vi "Periodic Tasks.vi"(8 "error in":errorcluster) -> ()   [LabVIEW 2018]
doc: "This VI runs in parallel to other tasks. It can contain as many user-defined periodic loops as you need. These can carry out PID or other sorts of timed response."
uses:
  <vilib>/Rock Robotics/WPI/ThirdParty/REV Robotics/SPARK MAX/Typedef/Spark MAX Faults.ctl
  <vilib>/Rock Robotics/WPI/ThirdParty/REV Robotics/SPARK MAX/Typedef/Spark MAX Limit Direction.ctl
  <vilib>/Rock Robotics/WPI/ThirdParty/REV Robotics/SPARK MAX/Typedef/Spark MAX Control Type.ctl
  <vilib>/Rock Robotics/WPI/Solenoid/WPI_SolenoidValue.ctl
  <vilib>/Rock Robotics/WPI/Utilities/WPI_GetSetVariantRefNum.vi
  <vilib>/Rock Robotics/WPI/Solenoid/WPI_SolenoidSetEnum.vi
  <vilib>/Rock Robotics/Network Tables/NT Write Boolean.vi
  <vilib>/Rock Robotics/Network Tables/NT Write Numeric Array.vi
  <vilib>/Rock Robotics/Network Tables/NT Write Boolean Array.vi
  <vilib>/Rock Robotics/Network Tables/NT Read Number.vi
  <vilib>/Rock Robotics/Network Tables/NT Write Number.vi
  <vilib>/addons/control/pid/pid.llb/PID (DBL).vi
  <vilib>/Rock Robotics/WPI/Solenoid/WPI_SolenoidGetEnum.vi
  <vilib>/addons/control/pid/NI_PID_pid.lvlib
panel:
  in  "setpoint":dbl format="%.2f"
  in  "cargoship":dbl=3.0 format="%#_13g"
  in  "rocket":dbl=4.699999999999999 format="%#_13g"
  in  "intake":dbl=10.65 format="%#_13g"
  out "Current":dbl=0.125
  out "Applied Output":dbl
  out "Set Point":i32=4
  out "x":dbl
  out "angle":dbl
  in  "PID Constants":T1={"P Gain"=0.08, "I Gain"=7e-05, "D Gain"=2.0, "F Gain"=0.0, "I Zone"=4.0, "Min Output"=-0.2, "Max Output"=0.05}
  in  "PID gains":T2={"proportional gain (Kc)"=0.01, "integral time (Ti, min)"=0.006, "derivative time (Td, min)"=0.0} {"derivative time (Td, min)" format="%.3f"; "integral time (Ti, min)" format="%.3f"; "proportional gain (Kc)" format="%.3f"}
  out "output":dbl=0.041618055988639956 format="%.2f"
  out "Direction":bool
  out "Turret Encoder":dbl=0.75
  out "Faults":T3={"Hard Limit Rev"=FALSE, "Hard Limit Fwd"=TRUE, "Soft Limit Fwd"=FALSE, "Soft Limit Rev"=FALSE, "Other Fault"=FALSE, "DRV Fault"=FALSE, "Has Reset?"=FALSE, "CAN RX"=FALSE, "CAN TX"=FALSE, "EEPROM CRC"=FALSE, "Stall"=FALSE, "Sensor Fault"=FALSE, "Motor Type Fault"=FALSE, "IWDT Reset"=FALSE, "Over Current"=FALSE, "Brownout"=FALSE}
  out "Sticky Faults":T3={"Hard Limit Rev"=FALSE, "Hard Limit Fwd"=FALSE, "Soft Limit Fwd"=FALSE, "Soft Limit Rev"=FALSE, "Other Fault"=FALSE, "DRV Fault"=FALSE, "Has Reset?"=FALSE, "CAN RX"=FALSE, "CAN TX"=TRUE, "EEPROM CRC"=FALSE, "Stall"=FALSE, "Sensor Fault"=FALSE, "Motor Type Fault"=FALSE, "IWDT Reset"=FALSE, "Over Current"=FALSE, "Brownout"=FALSE}
  out "Left Motor RPM":dbl
  out "Left Motor Rotations":dbl=10.976247787475586 format="%#_6p"
  # "SPARX MAX/ARM"
  # "SPARX/TURRET"
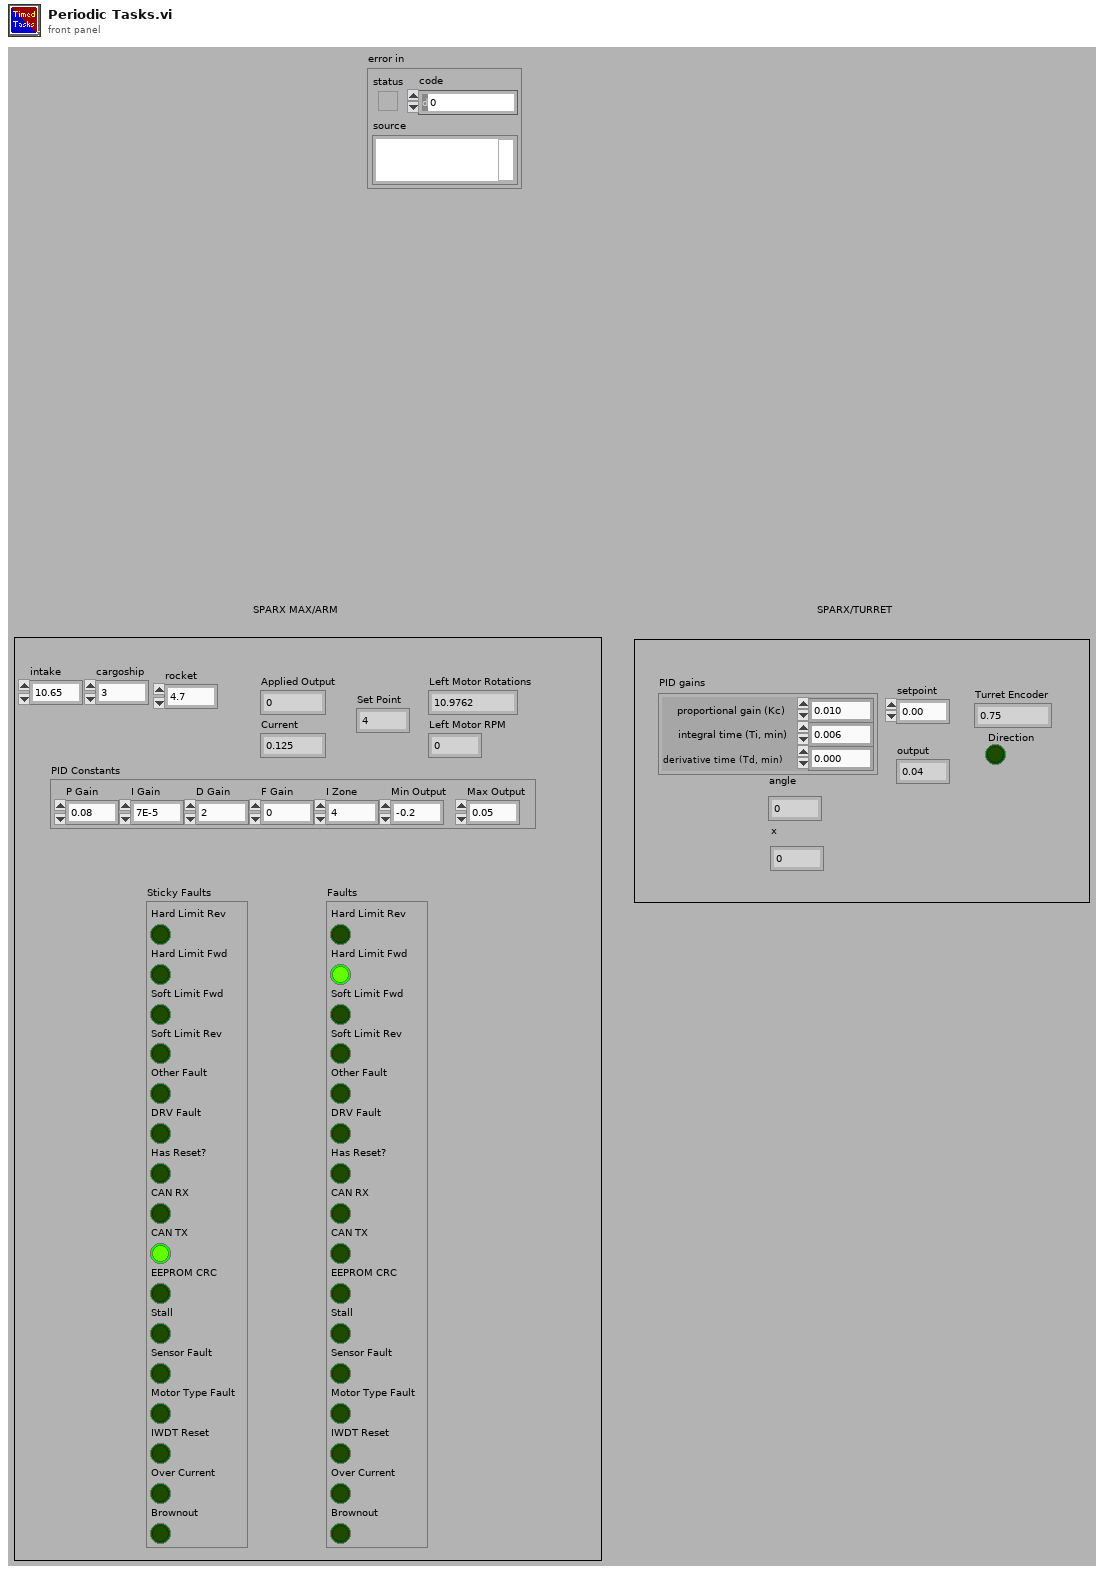
[diagram p1: front panel]
types:
  T1 = cluster{"P Gain":dbl, "I Gain":dbl, "D Gain":dbl, "F Gain":dbl, "I Zone":dbl, "Min Output":dbl, "Max Output":dbl}
  T2 = cluster{"proportional gain (Kc)":dbl, "integral time (Ti, min)":dbl, "derivative time (Td, min)":dbl}
  T3 = typedef "Spark MAX Faults.ctl" = cluster{"Hard Limit Rev":bool, "Hard Limit Fwd":bool, "Soft Limit Fwd":bool, "Soft Limit Rev":bool, "Other Fault":bool, "DRV Fault":bool, "Has Reset?":bool, "CAN RX":bool, "CAN TX":bool, "EEPROM CRC":bool, "Stall":bool, "Sensor Fault":bool, "Motor Type Fault":bool, "IWDT Reset":bool, "Over Current":bool, "Brownout":bool}
  T4 = typedef "WPI_JoystickDevRef.ctl" = cluster{"Device":T5}
  T5 = typedef "WPI_JoystickDeviceEnum.ctl" = enum16{"USB 0", "USB 1", "USB 2", "USB 3", "USB 4", "USB 5"}
  T6 = typedef "WPI_RobotDriveDevRef.ctl" = cluster{"DevStatus":errorcluster, "Motors[]":T7[], "Square Inputs":bool, "Max Output":dbl}
  T7 = typedef "WPI_MotorControlDeviceRef.ctl" = cluster{"DeviceStatus":errorcluster, "Type":T8, "PWM":cluster{"PWM Channel":T9, "DeadBand":T10}, "CAN":cluster{"Device Number":u8, "SetOutput VI Ref":variant, "GetOutput VI Ref":variant, "Enable VI Ref":variant, "Disable VI Ref":variant, "Data":variant}, "Invert":bool, "DIO PWM":cluster{"PWM \"Enable\" Channel":T9, "DIOChannel":T11, "PWM Rate":dbl}}
  T8 = typedef "WPI_MotorControlType.ctl" = enum16{"PWM", "CAN", "DIO PWM"}
  T9 = typedef "FPGA_DIOPWMChannel.ctl" = enum8{"PWM 0", "PWM 1", "PWM 2", "PWM 3", "PWM 4", "PWM 5", "PWM 6", "PWM 7", "PWM 8", "PWM 9", "PWM MXP 0", "PWM MXP 1", "PWM MXP 2", "PWM MXP 3", "PWM MXP 4", "PWM MXP 5", "PWM MXP 6", "PWM MXP 7", "PWM MXP 8", "PWM MXP 9", "Invalid"}
  T10 = typedef "WPI_PWMDeadband.ctl" = cluster{"Name":string, "maxPositivePwm":i32, "minPositivePwm":i32, "centerPwm":i32, "maxNegativePwm":i32, "minNegativePwm":i32, "angularRange":u16}
  T11 = typedef "FPGA_DIOChannel.ctl" = enum8{"DIO 0", "DIO 1", "DIO 2", "DIO 3", "DIO 4", "DIO 5", "DIO 6", "DIO 7", "DIO 8", "DIO 9", "DIO MXP 0", "DIO MXP 1", "DIO MXP 2", "DIO MXP 3", "DIO MXP 4", "DIO MXP 5", "DIO MXP 6", "DIO MXP 7", "DIO MXP 8", "DIO MXP 9", "DIO MXP 10", "DIO MXP 11", "DIO MXP 12", "DIO MXP 13", "DIO MXP 14", "DIO MXP 15", "SPI Port CS1", "SPI Port CS2", "SPI Port CS3", "SPI Port MISO", "SPI Port MOSI", "Invalid"}
  T12 = typedef "Spark MAX Control Type.ctl" = enum16{"Percent VBus", "Voltage", "Velocity", "Position", "Smart Motion", "Current", "Smart Velocity"}
  T13 = typedef "Spark MAX Limit Direction.ctl" = enum16{"Forward Limit", "Reverse Limit"}
  T14 = typedef "WPI_EncoderDevRef.ctl" = cluster{"DevStatus":errorcluster, "EncoderIndex":T15, "CounterIndex":T16, "DistancePerCount":dbl, "Decoding Type":T17}
  T15 = typedef "FPGA_EncoderIdx.ctl" = enum8{"Enc 0", "Enc 1", "Enc 2", "Enc 3", "Enc 4", "Enc 5", "Enc 6", "Enc 7", "Invalid"}
  T16 = typedef "FPGA_CounterCtrSystemIndex.ctl" = enum8{"Ctr 0", "Ctr 1", "Ctr 2", "Ctr 3", "Ctr 4", "Ctr 5", "Ctr 6", "Ctr 7", "Invalid"}
  T17 = typedef "WPI_EncoderType.ctl" = enum16{"1x", "2x", "4x"}
  T18 = typedef "WPI_SwitchDevRef.ctl" = cluster{"DevStatus":errorcluster, "DIO Channel":T11, "CntIndex":T16, "Normally Closed":bool}
  T19 = typedef "WPI_SolenoidValue.ctl" = enum16{"Off", "On", "Forward", "Reverse"}
  T20 = typedef "WPI_SolenoidDevRef.ctl" = cluster{"DevStatus":errorcluster, "Pneumatics Control Module":u8, "Forward Solenoid Channel":T21, "Reverse Solenoid Channel":T21}
  T21 = typedef "WPI_SolenoidChannel.ctl" = enum8{"Solenoid 0", "Solenoid 1", "Solenoid 2", "Solenoid 3", "Solenoid 4", "Solenoid 5", "Solenoid 6", "Solenoid 7", "Invalid"}
  T22 = typedef "WPI_DigitalInputDevRef.ctl" = cluster{"DevStatus":errorcluster, "DIO Channel":T11}
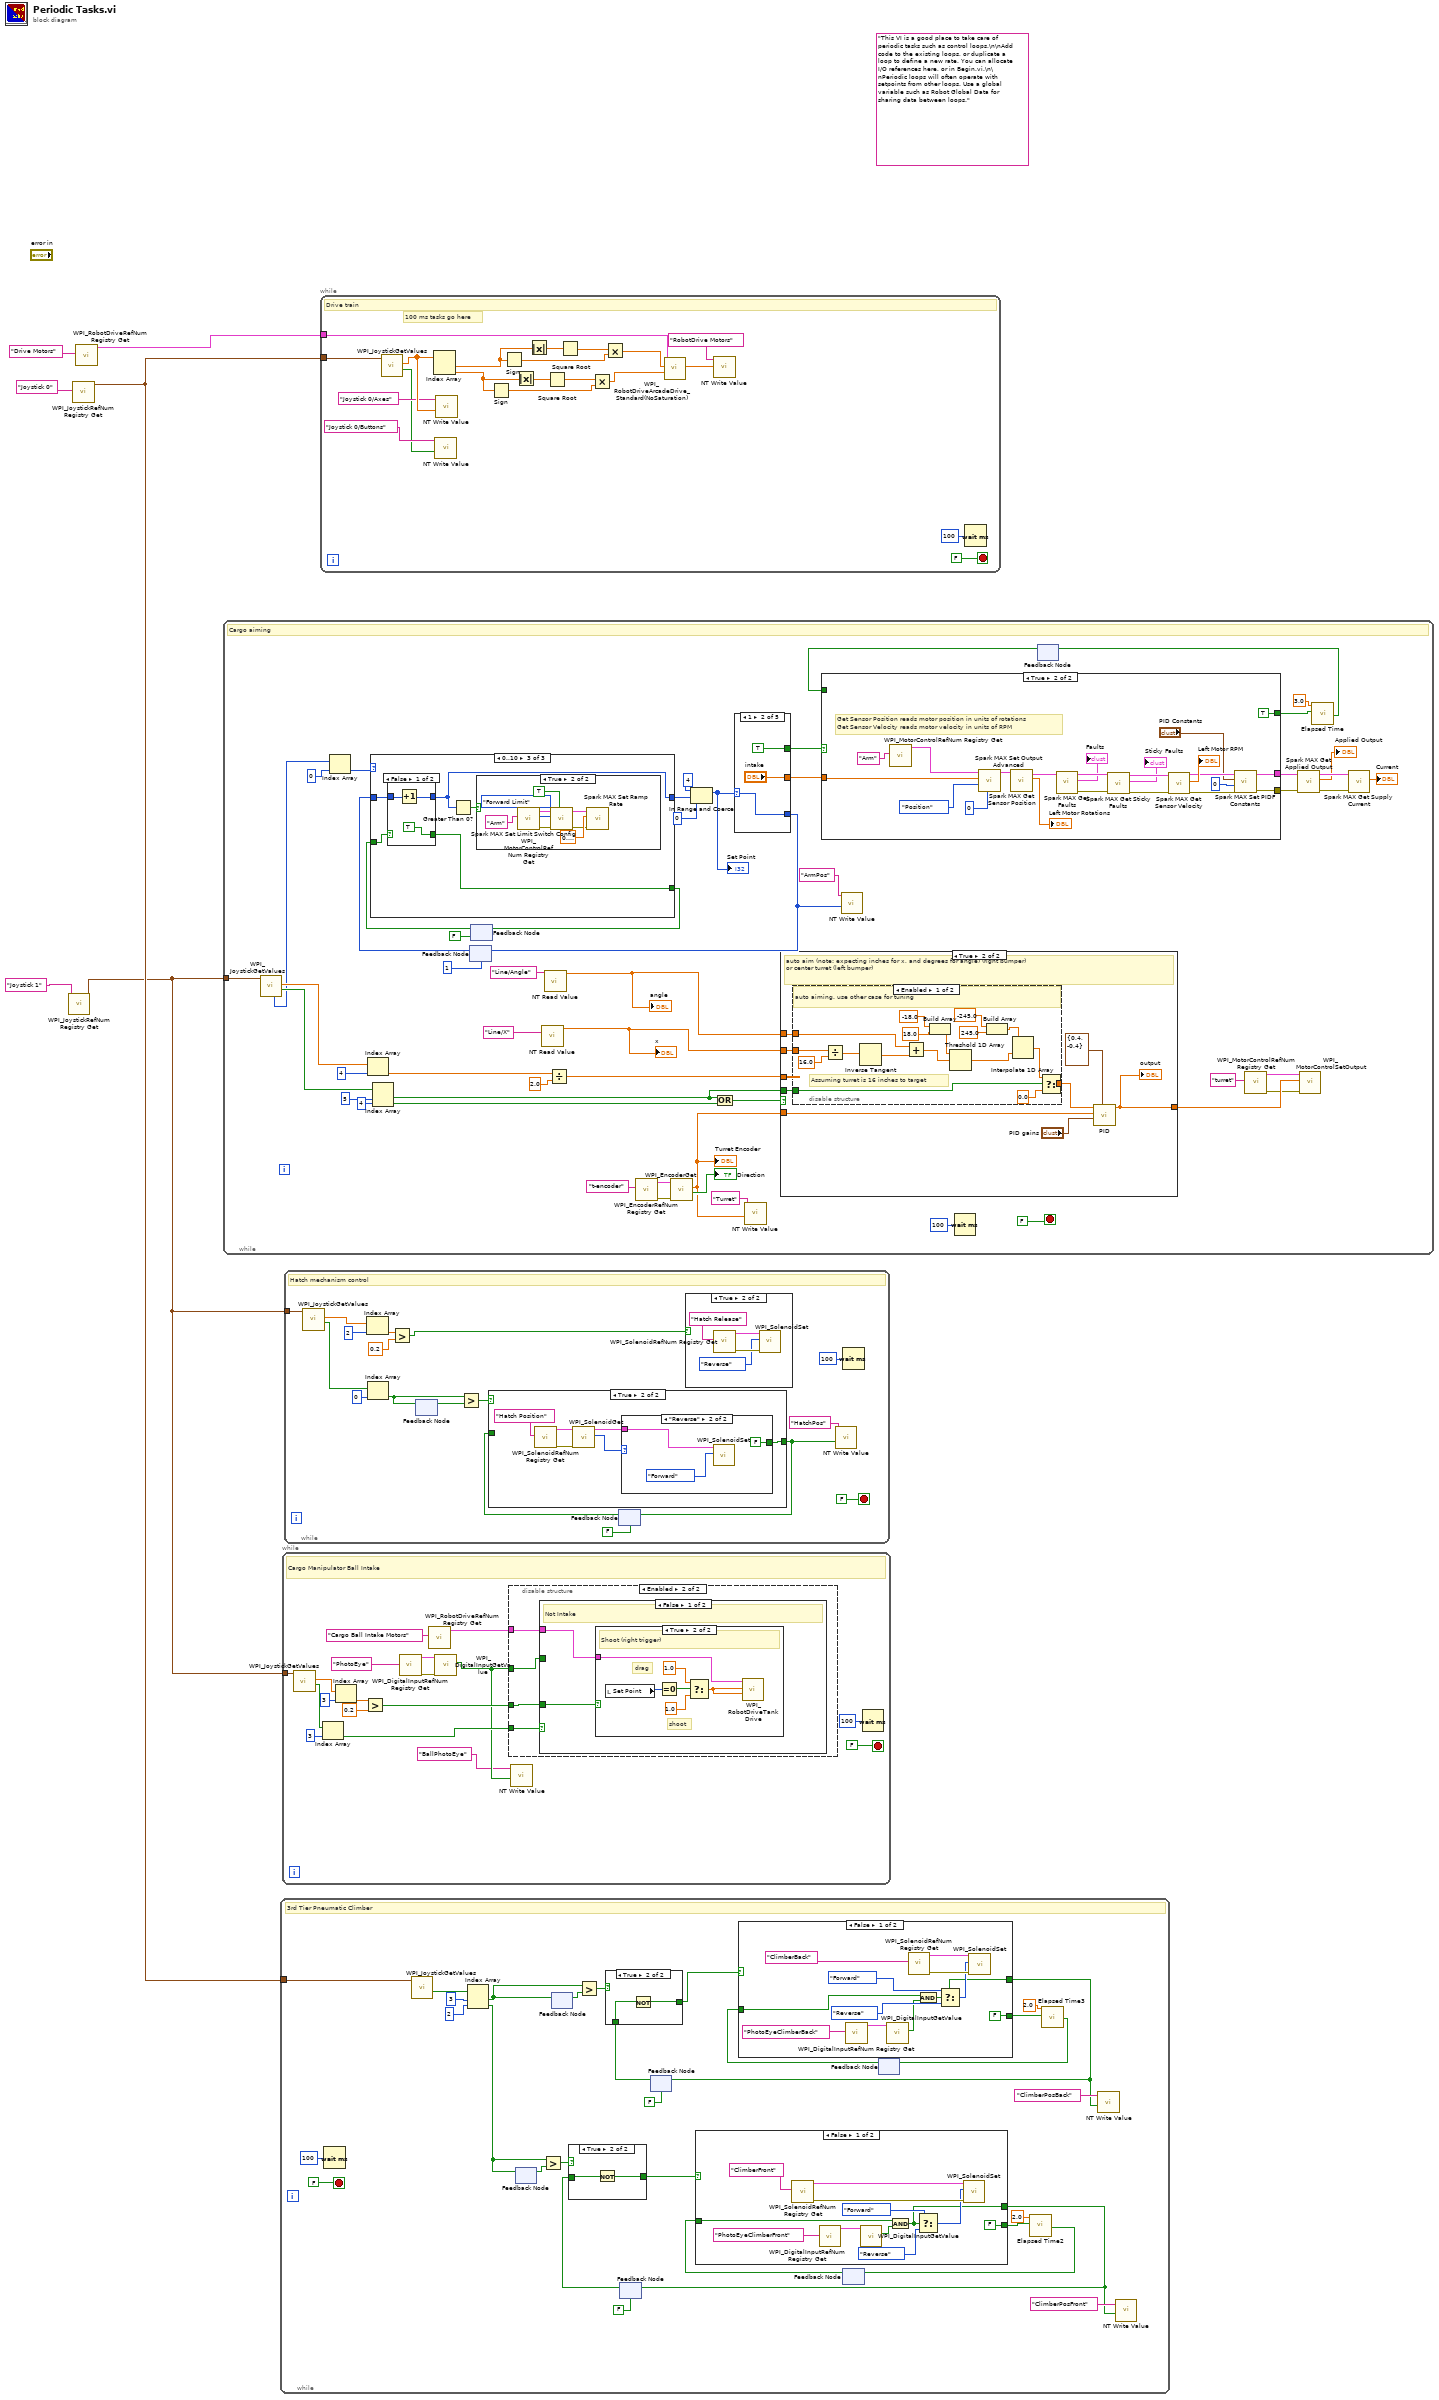
[diagram p0: block diagram]
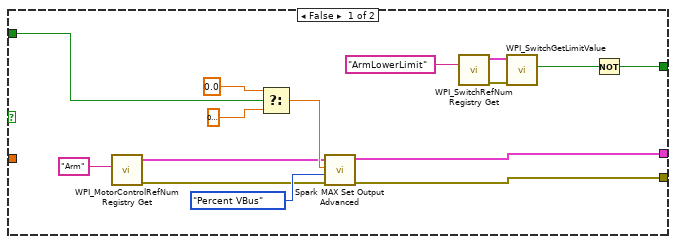
[diagram p2: hidden frame]
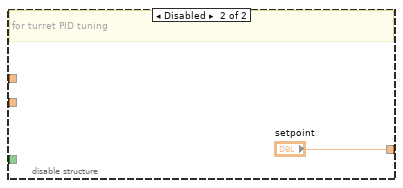
[diagram p4: hidden frame]
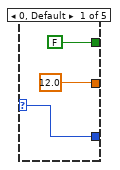
[diagram p5: hidden frame]
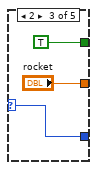
[diagram p6: hidden frame]
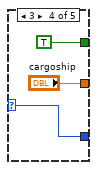
[diagram p7: hidden frame]
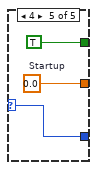
[diagram p8: hidden frame]
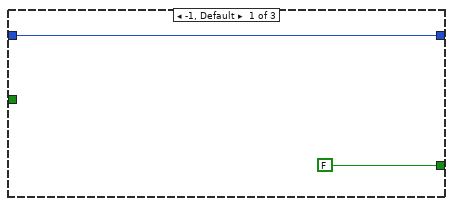
[diagram p9: hidden frame]
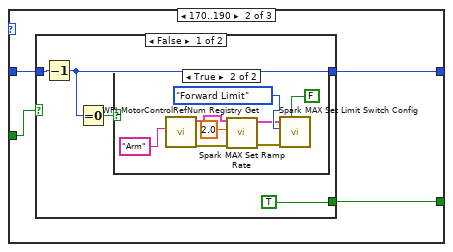
[diagram p10: hidden frame]
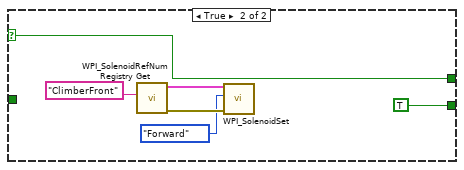
[diagram p16: hidden frame]
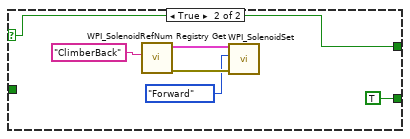
[diagram p18: hidden frame]
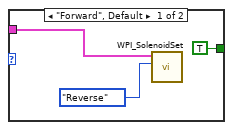
[diagram p20: hidden frame]
diagram:
  (unwired) "This VI is a good place to take care of periodic tasks such as control loops.\n\nAdd code to the existing loops, or duplicate a loop to define a new rate. You can allocate I/O references here, or in Begin.vi.\n\nPeriodic loops will often operate with setpoints from other loops. Use a global variable such as Robot Global Data for sharing data between loops."
  n1 = call <vilib>:"WPI_JoystickRefNum Registry Get.vi"("refnum name"="Joystick 1") -> ("JoystickDevRef"=w1:T4)  [unwired: 1 in, 9 out]
  n2 = call <vilib>:"WPI_JoystickRefNum Registry Get.vi"("refnum name"="Joystick 0") -> ("JoystickDevRef"=w2:T4)  [unwired: 1 in, 9 out]
  n3 = call <vilib>:"WPI_RobotDriveRefNum Registry Get.vi"("refnum name"="Drive Motors") -> ("RobotDriveDevRef"=w4:T6)  [unwired: 1 in, 9 out]
  n4 = while {
    tunnel: w1 -> [w54]
    stop <- FALSE stop-if-true
    # "Cargo aiming"
    n5 = call <vilib>:"WPI_JoystickGetValues.vi"("JoystickDevRef"=w54) -> ("Buttons"=w51:bool[], "Axes"=w53:dbl[], "POVs"=w47:i16[])  [unwired: 6 in, 2 out]
    n6 = Index Array(array=w47, index=0) -> (element=w45:i16)
    n7 = Index Array(array=w53, index=4) -> (element=w42:dbl)
    n8 = Index Array(array=w51, index #1=5 ("index"), index #2=4 ("index")) -> (element #1=w22:bool, element #2=w23:bool)
    n9 = feedback #1(1) -> (w44:i32)
    n10 = feedback #2(FALSE) -> (w28:bool)
    n11 = case shown="0..10" w45 {
      tunnel: w28 -> [_ w143 w163]
      tunnel: [FALSE w142 w162] -> w29
      tunnel: w44 -> [w140 w145 w164]
      tunnel: [w140 w144 w161] -> w27
      frame -1, Default {
      }
      frame 170..190 {
        n12 = case shown="False" w143 {
          selector: w143 -> [_ w158]
          tunnel: w145 -> [w149 w159]
          tunnel: [w146 w159] -> w144
          tunnel: [TRUE w158] -> w142
          frame False {
            n13 = Decrement(x=w149) -> (x-1=w146:i32)
            n14 = Equal To 0?(x=w146) -> (x = 0?=w147:bool)
            n15 = case shown="True" w147 {
              frame False {
              }
              frame True {
                n16 = call <vilib>:"WPI_MotorControlRefNum Registry Get.vi"("refnum name"="Arm") -> ("error out"=w150:errorcluster, "MotorControlDevRef"=w153:T7)  [unwired: 9 in]
                n17 = call <vilib>:"Spark MAX Set Ramp Rate.vi"("error in (no error)"=w150, "Seconds from neutral to full (0)"=sgl 2.0, "MotorControlDeviceRef in"=w153) -> ("error out"=w151:errorcluster, "MotorControlDeviceRef"=w152:T7)  [unwired: 7 in]
                n18 = call <vilib>:"Spark MAX Set Limit Switch Config.vi"("Enabled? (T)"=FALSE, "error in (no error)"=w151, "Limit Switch"=Spark_MAX_Limit_Direction."Forward Limit", "MotorControlDeviceRef in"=w152) -> ()  [unwired: 6 in, 2 out]
              }
            }
          }
          frame True {
          }
        }
      }
      frame 0..10 {
        n19 = case shown="False" w163 {
          selector: w163 -> [_ w177]
          tunnel: w164 -> [w175 w176]
          tunnel: [w174 w176] -> w161
          tunnel: [TRUE w177] -> w162
          frame False {
            n20 = Increment(x=w175) -> (x+1=w174:i32)
          }
          frame True {
          }
        }
        n21 = Greater Than 0?(x=w161) -> (x > 0?=w160:bool)
        n22 = case shown="True" w160 {
          frame False {
          }
          frame True {
            n23 = call <vilib>:"WPI_MotorControlRefNum Registry Get.vi"("refnum name"="Arm") -> ("error out"=w171:errorcluster, "MotorControlDevRef"=w170:T7)  [unwired: 9 in]
            n24 = call <vilib>:"Spark MAX Set Limit Switch Config.vi"("Enabled? (T)"=TRUE, "error in (no error)"=w171, "Limit Switch"=Spark_MAX_Limit_Direction."Forward Limit", "MotorControlDeviceRef in"=w170) -> ("error out"=w166:errorcluster, "MotorControlDeviceRef out"=w165:T7)  [unwired: 6 in]
            n25 = call <vilib>:"Spark MAX Set Ramp Rate.vi"("error in (no error)"=w166, "Seconds from neutral to full (0)"=sgl 0.1, "MotorControlDeviceRef in"=w165) -> ()  [unwired: 7 in, 2 out]
          }
        }
      }
    }
    n26 = feedback-in #2(w29) -> ()
    n27 = call-poly <vilib>:"NT Read Value.vi"("Name"="Line/X") -> ("Numeric"=w10:dbl)  [unwired: 9 in, 1 out]
    "x" <- w10
    n28 = call-poly <vilib>:"NT Read Value.vi"("Name"="Line/Angle") -> ("Numeric"=w9:dbl)  [unwired: 9 in, 1 out]
    "angle" <- w9
    n29 = Divide(x=w42, y=2.0) -> (x/y=w33:dbl)
    n30 = call <vilib>:"WPI_EncoderRefNum Registry Get.vi"("refnum name"="t-encoder") -> ("error out"=w59:errorcluster, "EncoderDevRef"=w58:T14)  [unwired: 9 in]
    n31 = call <vilib>:"WPI_EncoderGet.vi"("error in (no error)"=w59, "EncoderDevRef"=w58) -> ("Direction"=→"Direction":bool, "Distance"=w7:dbl)  [unwired: 4 in, 4 out]
    "Turret Encoder" <- w7
    n32 = In Range and Coerce(upper limit=4, x=w27, lower limit=0) -> (coerced(x)=w25:i32)  [unwired: 1 out]
    "Set Point" <- w25
    n33 = Or(x=w22, y=w23) -> (x .or. y?=w24:bool)
    n34 = case shown="1" w25 {
      selector: w25 -> [w127 w129 w132 w135 w138]
      tunnel: [12.0 "intake" "rocket" "cargoship" w139] -> w41
      tunnel: [w127 w129 w132 w135 w138] -> w38
      tunnel: [FALSE TRUE TRUE TRUE TRUE] -> w40
      frame 0, Default {
      }
      frame 1 {
      }
      frame 2 {
      }
      frame 3 {
      }
      frame 4 {
        w139 = 0.0  # Startup
      }
    }
    n35 = feedback-in #1(w38) -> ()
    n36 = call-poly <vilib>:"NT Write Value.vi"("Numeric"=w7, "Name"="Turret") -> ()  [unwired: 9 in, 1 out]
    n37 = case shown="True" w24 {
      tunnel: w9 -> [_ w101]
      tunnel: w10 -> [_ w102]
      tunnel: w33 -> [w98 _]
      tunnel: [w98 w103] -> w39
      tunnel: w7 -> [_ w104]
      tunnel: w22 -> [_ w100]
      frame False {
        # "manual control"
      }
      frame True {
        # "auto aim (note: expecting inches for x, and degrees for angle) (right bumper)\nor center turret (left bumper)"
        n38 = disable-structure shown="Enabled" {
          disable-tunnel: w102 -> [w123 _]
          disable-tunnel: w101 -> [w121 _]
          disable-tunnel: w100 -> [w108 _]
          disable-tunnel: [w107 "setpoint"] -> w99
          frame Enabled {
            # "Assuming turret is 16 inches to target"
            # "auto aiming. use other case for tuning"
            n39 = Divide(x=w123, y=16.0) -> (x/y=w112:dbl)
            n40 = Inverse Tangent(1:w112) -> (0:w111:dbl)
            n41 = Add(x=w121, y=w111) -> (x+y=w115:dbl)
            n42 = Build Array(-18.0 ("lower limit"), 18.0 ("upper limit")) -> (w116:dbl[])
            n43 = Threshold 1D Array(2:w115, 3:w116) -> (0:w113:dbl)  [unwired: 1 in]
            n44 = Build Array(-245.0 ("lower limit"), 245.0 ("upper limit")) -> (w114:dbl[])
            n45 = Interpolate 1D Array(1:w113, 2:w114) -> (0:w110:dbl)
            n46 = Select(t=w110, s=w108, f=0.0) -> (s? t:f=w107:dbl)
          }
          frame Disabled {
            # "for turret PID tuning"
          }
        }
        n47 = call-poly <vilib>:"PID.vi"("output range"=cluster{"output high":dbl, "output low":dbl} {"output high"=0.4, "output low"=-0.4}, "PID gains"="PID gains", "process variable"=w104, "setpoint"=w99) -> ("output"=w103:dbl)  [unwired: 6 in, 1 out]
        "output" <- w103
      }
    }
    n48 = call-poly <vilib>:"NT Write Value.vi"("Numeric"=w38, "Name"="ArmPos") -> ()  [unwired: 9 in, 1 out]
    n49 = Wait (ms)(milliseconds to wait=u32 100) -> ()  [unwired: 1 out]
    n50 = feedback #3() -> (w12:bool)  [unwired: 1 in]
    n51 = case shown="True" w40 {
      tunnel: w41 -> [_ w79]
      tunnel: [w68 w77] -> w16
      tunnel: [w67 w78] -> w15
      tunnel: w12 -> [w66 _]
      tunnel: [w65 TRUE] -> w11
      frame False {
        n52 = call <vilib>:"WPI_MotorControlRefNum Registry Get.vi"("refnum name"="Arm") -> ("error out"=w69:errorcluster, "MotorControlDevRef"=w70:T7)  [unwired: 9 in]
        n53 = Select(t=0.0, s=w66, f=0.9999999999999999 ("Setpoint")) -> (s? t:f=w71:dbl)
        n54 = call <vilib>:"Spark MAX Set Output Advanced.vi"("error in (no error)"=w69, "Control Mode"=Spark_MAX_Control_Type."Percent VBus", "Setpoint"=w71, "MotorControlDevRef"=w70) -> ("error out"=w68:errorcluster, "MotorControlDevRef"=w67:T7)  [unwired: 6 in]
        n55 = call <vilib>:"WPI_SwitchRefNum Registry Get.vi"("refnum name"="ArmLowerLimit") -> ("error out"=w63:errorcluster, "SwitchDevRef"=w64:T18)  [unwired: 9 in]
        n56 = call <vilib>:"WPI_SwitchGetLimitValue.vi"("error in (no error)"=w63, "SwitchDevRef"=w64) -> ("Switch Pressed"=w61:bool)  [unwired: 7 in, 2 out]
        n57 = Not(x=w61) -> (.not. x?=w65:bool)
      }
      frame True {
        # "Get Sensor Position reads motor position in units of rotations\nGet Sensor Velocity reads motor velocity in units of RPM"
        n58 = call <vilib>:"WPI_MotorControlRefNum Registry Get.vi"("refnum name"="Arm") -> ("MotorControlDevRef"=w81:T7)  [unwired: 9 in, 1 out]
        n59 = call <vilib>:"Spark MAX Set Output Advanced.vi"("PIDF Slot (0)"=0, "Control Mode"=Spark_MAX_Control_Type."Position", "Setpoint"=w79, "MotorControlDevRef"=w81) -> ("MotorControlDevRef"=w95:T7)  [unwired: 6 in, 1 out]
        n60 = call <vilib>:"Spark MAX Get Sensor Position.vi"("MotorControlDevRef in"=w95) -> ("Sensor Position"=→"Left Motor Rotations":dbl, "MotorControlDevRef out"=w93:T7)  [unwired: 7 in, 2 out]
        n61 = call <vilib>:"Spark MAX Get Faults.vi"("MotorControlDevRef in"=w93) -> ("error out"=w92:errorcluster, "Faults"=→"Faults":T3, "MotorControlDevRef out"=w91:T7)  [unwired: 7 in, 1 out]
        n62 = call <vilib>:"Spark MAX Get Sticky Faults.vi"("error in (no error)"=w92, "MotorControlDevRef in"=w91) -> ("error out"=w89:errorcluster, "Sticky Faults"=→"Sticky Faults":T3, "MotorControlDevRef out"=w90:T7)  [unwired: 6 in, 1 out]
        n63 = call <vilib>:"Spark MAX Get Sensor Velocity.vi"("error in (no error)"=w89, "MotorControlDevRef in"=w90) -> ("error out"=w84:errorcluster, "Sensor Velocity"=→"Left Motor RPM":dbl, "MotorControlDevRef out"=w85:T7)  [unwired: 6 in, 1 out]
        n64 = call <vilib>:"Spark MAX Set PIDF Constants.vi"("error in"=w84, "PIDF Slot"=0, "PID Constants"="PID Constants", "MotorControlDeviceRef"=w85) -> ("error out"=w77:errorcluster, "MotorControlDeviceRef"=w78:T7)  [unwired: 6 in]
      }
    }
    n65 = call <vilib>:"WPI_MotorControlRefNum Registry Get.vi"("refnum name"="turret") -> ("error out"=w35:errorcluster, "MotorControlDevRef"=w34:T7)  [unwired: 9 in]
    n66 = call <vilib>:"Spark MAX Get Applied Output.vi"("error in (no error)"=w16, "MotorControlDevRef in"=w15) -> ("error out"=w18:errorcluster, "Applied Output"=→"Applied Output":dbl, "MotorControlDevRef out"=w19:T7)  [unwired: 6 in, 1 out]
    n67 = call <vilib>:"WPI_MotorControlSetOutput.vi"("error in (no error)"=w35, "Output"=w39, "MotorControlDevRef"=w34) -> ()  [unwired: 6 in, 3 out]
    n68 = call "Elapsed Time"("Time Target (s)"=3.0, "Reset"=w11) -> ("Time has Elapsed"=w13:bool)  [unwired: 10 in, 7 out]
    n69 = feedback-in #3(w13) -> ()
    n70 = call <vilib>:"Spark MAX Get Supply Current.vi"("error in (no error)"=w18, "MotorControlDevRef in"=w19) -> ("Current"=→"Current":dbl)  [unwired: 6 in, 3 out]
  }
  n71 = while {
    tunnel: w2 -> [w205]
    stop <- FALSE stop-if-true
    # "3rd Tier Pneumatic Climber"
    n72 = Wait (ms)(milliseconds to wait=u32 100) -> ()  [unwired: 1 out]
    n73 = call <vilib>:"WPI_JoystickGetValues.vi"("JoystickDevRef"=w205) -> ("Buttons"=w204:bool[])  [unwired: 6 in, 4 out]
    n74 = Index Array(array=w204, index #1=3 ("index"), index #2=2 ("index")) -> (element #1=w199:bool, element #2=w190:bool)
    n75 = feedback #4() -> (w193:bool)  [unwired: 1 in]
    n76 = feedback-in #4(w190) -> ()
    n77 = Greater?(x=w190, y=w193) -> (0:w192:bool)
    n78 = feedback #5() -> (w201:bool)  [unwired: 1 in]
    n79 = feedback-in #5(w199) -> ()
    n80 = Greater?(x=w199, y=w201) -> (0:w200:bool)
    n81 = feedback #6(FALSE) -> (w191:bool)
    n82 = case shown="True" w192 {
      tunnel: w191 -> [w208 w210]
      tunnel: [w208 w209] -> w188
      frame False {
      }
      frame True {
        n83 = Not(x=w210) -> (.not. x?=w209:bool)
      }
    }
    n84 = feedback #7(FALSE) -> (w198:bool)
    n85 = case shown="True" w200 {
      tunnel: w198 -> [w229 w231]
      tunnel: [w229 w230] -> w197
      frame False {
      }
      frame True {
        n86 = Not(x=w231) -> (.not. x?=w230:bool)
      }
    }
    n87 = feedback #8() -> (w185:bool)  [unwired: 1 in]
    n88 = case shown="False" w188 {
      selector: w188 -> [_ w223]
      tunnel: [FALSE TRUE] -> w187
      tunnel: w185 -> [w216 _]
      tunnel: [w211 w223] -> w183
      frame False {
        n89 = call <vilib>:"WPI_SolenoidRefNum Registry Get.vi"("refnum name"="ClimberFront") -> ("error out"=w221:errorcluster, "SolenoidDevRef"=w222:T20)  [unwired: 9 in]
        n90 = call <vilib>:"WPI_DigitalInputRefNum Registry Get.vi"("refnum name"="PhotoEyeClimberFront") -> ("DigitalInputDevRef"=w219:T22)  [unwired: 9 in, 1 out]
        n91 = call <vilib>:"WPI_DigitalInputGetValue.vi"("DigitalInputDevRef"=w219) -> ("Value"=w217:bool)  [unwired: 8 in, 2 out]
        n92 = And(x=w216, y=w217) -> (x .and. y?=w211:bool)
        n93 = Select(t=WPI_SolenoidValue."Forward", s=w211, f=WPI_SolenoidValue."Reverse" ("Value")) -> (s? t:f=w213:T19)
        n94 = call-poly <vilib>:"WPI_SolenoidSet.vi"("error in (no error)"=w221, "Value"=w213, "SolenoidDevRef"=w222) -> ()  [unwired: 7 in, 2 out]
      }
      frame True {
        n95 = call <vilib>:"WPI_SolenoidRefNum Registry Get.vi"("refnum name"="ClimberFront") -> ("error out"=w227:errorcluster, "SolenoidDevRef"=w228:T20)  [unwired: 9 in]
        n96 = call-poly <vilib>:"WPI_SolenoidSet.vi"("error in (no error)"=w227, "Value"=WPI_SolenoidValue."Forward", "SolenoidDevRef"=w228) -> ()  [unwired: 7 in, 2 out]
      }
    }
    n97 = feedback-in #6(w183) -> ()
    n98 = feedback #9() -> (w179:bool)  [unwired: 1 in]
    n99 = case shown="False" w197 {
      selector: w197 -> [_ w244]
      tunnel: [FALSE TRUE] -> w181
      tunnel: w179 -> [w234 _]
      tunnel: [w232 w244] -> w178
      frame False {
        n100 = call <vilib>:"WPI_DigitalInputRefNum Registry Get.vi"("refnum name"="PhotoEyeClimberBack") -> ("DigitalInputDevRef"=w240:T22)  [unwired: 9 in, 1 out]
        n101 = call <vilib>:"WPI_DigitalInputGetValue.vi"("DigitalInputDevRef"=w240) -> ("Value"=w235:bool)  [unwired: 8 in, 2 out]
        n102 = call <vilib>:"WPI_SolenoidRefNum Registry Get.vi"("refnum name"="ClimberBack") -> ("error out"=w242:errorcluster, "SolenoidDevRef"=w243:T20)  [unwired: 9 in]
        n103 = And(x=w234, y=w235) -> (x .and. y?=w232:bool)
        n104 = Select(t=WPI_SolenoidValue."Forward", s=w232, f=WPI_SolenoidValue."Reverse" ("Value")) -> (s? t:f=w236:T19)
        n105 = call-poly <vilib>:"WPI_SolenoidSet.vi"("error in (no error)"=w242, "Value"=w236, "SolenoidDevRef"=w243) -> ()  [unwired: 7 in, 2 out]
      }
      frame True {
        n106 = call <vilib>:"WPI_SolenoidRefNum Registry Get.vi"("refnum name"="ClimberBack") -> ("error out"=w249:errorcluster, "SolenoidDevRef"=w248:T20)  [unwired: 9 in]
        n107 = call-poly <vilib>:"WPI_SolenoidSet.vi"("error in (no error)"=w249, "Value"=WPI_SolenoidValue."Forward", "SolenoidDevRef"=w248) -> ()  [unwired: 7 in, 2 out]
      }
    }
    n108 = feedback-in #7(w178) -> ()
    n109 = call "Elapsed Time2"("Time Target (s)"=2.0, "Reset"=w187) -> ("Time has Elapsed"=w186:bool)  [unwired: 10 in, 7 out]
    n110 = feedback-in #8(w186) -> ()
    n111 = call "Elapsed Time3"("Time Target (s)"=2.0, "Reset"=w181) -> ("Time has Elapsed"=w180:bool)  [unwired: 10 in, 7 out]
    n112 = feedback-in #9(w180) -> ()
    n113 = call-poly <vilib>:"NT Write Value.vi"("Boolean"=w178, "Name"="ClimberPosBack") -> ()  [unwired: 9 in, 1 out]
    n114 = call-poly <vilib>:"NT Write Value.vi"("Boolean"=w183, "Name"="ClimberPosFront") -> ()  [unwired: 9 in, 1 out]
  }
  n115 = while {
    tunnel: w1 -> [w264]
    stop <- FALSE stop-if-true
    # "Cargo Manipulator Ball Intake"
    n116 = call <vilib>:"WPI_JoystickGetValues.vi"("JoystickDevRef"=w264) -> ("Buttons"=w263:bool[], "Axes"=w260:dbl[])  [unwired: 6 in, 3 out]
    n117 = Index Array(array=w263, index=3) -> (element=w255:bool)
    n118 = Index Array(array=w260, index=3) -> (element=w258:dbl)
    n119 = Greater?(x=w258, y=0.2) -> (0:w256:bool)
    n120 = call <vilib>:"WPI_DigitalInputRefNum Registry Get.vi"("refnum name"="PhotoEye") -> ("error out"=w254:errorcluster, "DigitalInputDevRef"=w253:T22)  [unwired: 9 in]
    n121 = call <vilib>:"WPI_RobotDriveRefNum Registry Get.vi"("refnum name"="Cargo Ball Intake Motors") -> ("RobotDriveDevRef"=w261:T6)  [unwired: 9 in, 1 out]
    n122 = call <vilib>:"WPI_DigitalInputGetValue.vi"("error in (no error)"=w254, "DigitalInputDevRef"=w253) -> ("Value"=w251:bool)  [unwired: 7 in, 2 out]
    n123 = disable-structure shown="Enabled" {
      disable-tunnel: w261 -> [w271 w293]
      disable-tunnel: w256 -> [w270 w294]
      disable-tunnel: w255 -> [w269 w295]
      disable-tunnel: w251 -> [w268 w296]
      frame Disabled {
        n124 = case shown="False" w268 {
          tunnel: w269 -> [w274 _]
          tunnel: w270 -> [w273 w285]
          tunnel: w271 -> [w272 w286]
          frame False {
            n125 = case shown="False" w274 {
              tunnel: w273 -> [w276 _]
              tunnel: w272 -> [w275 w284]
              frame False {
                n126 = case shown="True" w276 {
                  tunnel: w275 -> [w277 w281]
                  frame False {
                    # "If neither button is pushed"
                    n127 = call <vilib>:"WPI_RobotDriveTankDrive.vi"("Right axis value"=0.0, "Left axis value"=0.0, "RobotDriveDevRef"=w277) -> ()  [unwired: 6 in, 3 out]
                  }
                  frame True {
                    w280 = 0.8 ("Left axis value")
                    # "If RT is pushed,\nand Y is released"
                    n128 = call <vilib>:"WPI_RobotDriveTankDrive.vi"("Right axis value"=w280, "Left axis value"=w280, "RobotDriveDevRef"=w281) -> ()  [unwired: 6 in, 3 out]
                  }
                }
              }
              frame True {
                # "If Y is pushed"
                n129 = call <vilib>:"WPI_RobotDriveTankDrive.vi"("Right axis value"=-0.6 ("RightSpeed"), "Left axis value"=-0.6 ("LeftSpeed"), "RobotDriveDevRef"=w284) -> ()  [unwired: 6 in, 3 out]
              }
            }
          }
          frame True {
            n130 = case shown="True" w285 {
              tunnel: w286 -> [w287 w290]
              frame False {
                # "If PhotoEye is high with no release button"
                n131 = call <vilib>:"WPI_RobotDriveTankDrive.vi"("Right axis value"=0.0 ("RightSpeed"), "Left axis value"=0.0 ("LeftSpeed"), "RobotDriveDevRef"=w287) -> ()  [unwired: 6 in, 3 out]
              }
              frame True {
                # "Release Ball if PhotoEye high and release\nbutton is pushed"
                n132 = call <vilib>:"WPI_RobotDriveTankDrive.vi"("Right axis value"=0.8 ("RightSpeed"), "Left axis value"=0.8 ("LeftSpeed"), "RobotDriveDevRef"=w290) -> ()  [unwired: 6 in, 3 out]
              }
            }
          }
        }
      }
      frame Enabled {
        n133 = case shown="False" w295 {
          tunnel: w296 -> [_ w308]
          tunnel: w294 -> [w298 _]
          tunnel: w293 -> [w297 w307]
          frame False {
            # "Not Intake"
            n134 = case shown="True" w298 {
              tunnel: w297 -> [w299 w301]
              frame False {
                w300 = 0.0 ("LeftSpeed")
                n135 = call <vilib>:"WPI_RobotDriveTankDrive.vi"("Right axis value"=w300, "Left axis value"=w300, "RobotDriveDevRef"=w299) -> ()  [unwired: 6 in, 3 out]
              }
              frame True {
                # "drag"
                # "shoot"
                # "Shoot (right trigger)"
                n136 = local read "Set Point"() -> (w306:i32)
                n137 = Equal To 0?(x=w306) -> (x = 0?=w305:bool)
                n138 = Select(t=1.0 ("LeftSpeed"), s=w305, f=1.0 ("LeftSpeed")) -> (s? t:f=w302:dbl)
                n139 = call <vilib>:"WPI_RobotDriveTankDrive.vi"("Right axis value"=w302, "Left axis value"=w302, "RobotDriveDevRef"=w301) -> ()  [unwired: 6 in, 3 out]
              }
            }
          }
          frame True {
            # "Intake? (Y)"
            n140 = Select(t=0.0, s=w308, f=-0.6 ("LeftSpeed")) -> (s? t:f=w309:dbl)
            n141 = call <vilib>:"WPI_RobotDriveTankDrive.vi"("Right axis value"=w309, "Left axis value"=w309, "RobotDriveDevRef"=w307) -> ()  [unwired: 6 in, 3 out]
          }
        }
      }
    }
    n142 = call-poly <vilib>:"NT Write Value.vi"("Boolean"=w251, "Name"="BallPhotoEye") -> ()  [unwired: 9 in, 1 out]
    n143 = Wait (ms)(milliseconds to wait=u32 100) -> ()  [unwired: 1 out]
  }
  n144 = while {
    tunnel: w1 -> [w328]
    stop <- FALSE stop-if-true
    # "Hatch mechanism control"
    n145 = call <vilib>:"WPI_JoystickGetValues.vi"("JoystickDevRef"=w328) -> ("Buttons"=w319:bool[], "Axes"=w324:dbl[])  [unwired: 6 in, 3 out]
    n146 = Index Array(array=w324, index=2) -> (element=w322:dbl)
    n147 = Index Array(array=w319, index=0) -> (element=w318:bool)
    n148 = Greater?(x=w322, y=0.2) -> (0:w321:bool)
    n149 = feedback #10() -> (w325:bool)  [unwired: 1 in]
    n150 = feedback-in #10(w318) -> ()
    n151 = Greater?(x=w318, y=w325) -> (0:w316:bool)
    n152 = feedback #11(FALSE) -> (w314:bool)
    n153 = case shown="True" w316 {
      tunnel: [w329 w330] -> w313
      tunnel: w314 -> [w329 _]
      frame False {
      }
      frame True {
        n154 = call <vilib>:"WPI_SolenoidRefNum Registry Get.vi"("refnum name"="Hatch Position") -> ("error out"=w334:errorcluster, "SolenoidDevRef"=w335:T20)  [unwired: 9 in]
        n155 = call-poly <vilib>:"WPI_SolenoidGet.vi"("error in (no error)"=w334, "SolenoidDevRef"=w335) -> ("Value"=w332:T19, "SolenoidDevRef"=w331:T20)  [unwired: 7 in, 1 out]
        n156 = case shown="\"Reverse\"" w332 {
          tunnel: w331 -> [w337 w340]
          tunnel: [TRUE FALSE] -> w330
          frame "Forward", Default {
            n157 = call-poly <vilib>:"WPI_SolenoidSet.vi"("Value"=WPI_SolenoidValue."Reverse", "SolenoidDevRef"=w337) -> ()  [unwired: 8 in, 2 out]
          }
          frame "Reverse" {
            n158 = call-poly <vilib>:"WPI_SolenoidSet.vi"("Value"=WPI_SolenoidValue."Forward", "SolenoidDevRef"=w340) -> ()  [unwired: 8 in, 2 out]
          }
        }
      }
    }
    n159 = feedback-in #11(w313) -> ()
    n160 = case shown="True" w321 {
      frame False {
        n161 = call <vilib>:"WPI_SolenoidRefNum Registry Get.vi"("refnum name"="Hatch Release") -> ("error out"=w343:errorcluster, "SolenoidDevRef"=w344:T20)  [unwired: 9 in]
        n162 = call-poly <vilib>:"WPI_SolenoidSet.vi"("error in (no error)"=w343, "Value"=WPI_SolenoidValue."Forward", "SolenoidDevRef"=w344) -> ()  [unwired: 7 in, 2 out]
      }
      frame True {
        n163 = call <vilib>:"WPI_SolenoidRefNum Registry Get.vi"("refnum name"="Hatch Release") -> ("error out"=w347:errorcluster, "SolenoidDevRef"=w348:T20)  [unwired: 9 in]
        n164 = call-poly <vilib>:"WPI_SolenoidSet.vi"("error in (no error)"=w347, "Value"=WPI_SolenoidValue."Reverse", "SolenoidDevRef"=w348) -> ()  [unwired: 7 in, 2 out]
      }
    }
    n165 = call-poly <vilib>:"NT Write Value.vi"("Boolean"=w313, "Name"="HatchPos") -> ()  [unwired: 9 in, 1 out]
    n166 = Wait (ms)(milliseconds to wait=u32 100) -> ()  [unwired: 1 out]
  }
  n167 = while {
    tunnel: w2 -> [w367]
    tunnel: w4 -> [w366]
    stop <- FALSE stop-if-true
    # "100 ms tasks go here"
    # "Drive train"
    n168 = call <vilib>:"WPI_JoystickGetValues.vi"("JoystickDevRef"=w367) -> ("Buttons"=w360:bool[], "Axes"=w363:dbl[])  [unwired: 6 in, 3 out]
    n169 = Index Array(array=w363) -> (element #1=w351:dbl, element #2=w352:dbl)  [unwired: 2 in]
    n170 = call-poly <vilib>:"NT Write Value.vi"("Boolean Array"=w360, "Name"="Joystick 0/Buttons") -> ()  [unwired: 9 in, 1 out]
    n171 = call-poly <vilib>:"NT Write Value.vi"("Numeric Array"=w363, "Name"="Joystick 0/Axes") -> ()  [unwired: 9 in, 1 out]
    n172 = Sign(1:w352) -> (0:w358:dbl)
    n173 = Sign(1:w351) -> (0:w354:dbl)
    n174 = Absolute Value(x=w352) -> (abs(x)=w359:dbl)
    n175 = Absolute Value(x=w351) -> (abs(x)=w355:dbl)
    n176 = Square Root(x=w359) -> (sqrt(x)=w357:dbl)
    n177 = Square Root(x=w355) -> (sqrt(x)=w353:dbl)
    n178 = Multiply(x=w357, y=w358) -> (x*y=w356:dbl)
    n179 = Multiply(x=w353, y=w354) -> (x*y=w350:dbl)
    n180 = call <vilib>:"WPI_RobotDriveArcadeDrive_Standard(NoSaturation).vi"("Y axis value"=w356, "X axis value"=w350, "RobotDriveDevRef"=w366) -> ("Motor Values"=w365:dbl[])  [unwired: 1 in, 7 out]
    n181 = call-poly <vilib>:"NT Write Value.vi"("Numeric Array"=w365, "Name"="RobotDrive Motors") -> ()  [unwired: 9 in, 1 out]
    n182 = Wait (ms)(milliseconds to wait=u32 100) -> ()  [unwired: 1 out]
  }
